vi "move2shoot Controller.vi"(8 "error in":errorcluster) -> ()   [LabVIEW 2015]
doc: "This VI executes continuously carrying out the current operation and responding to updates or new operations. It will often contain the timing or control code that is difficult to place directly in TeleOp. This VI generally opens all sensors and motors and isolates the rest of the robot code from knowing how the operations are carried out."
uses:
  move2shoot Setpoints.ctl
  move2shoot Operations.ctl
  <vilib>/Rock Robotics/WPI/SafetyOutput/WPI_SafetyOutputConfigMenu.ctl
  <vilib>/Rock Robotics/SystemInterfaces/AI/FPGA_AIChannel.ctl
  <vilib>/Rock Robotics/WPI/MotorControl/WPI_MotorControlOpenCANTalonSRX.vi
  Vision/distance.vi
  <vilib>/addons/control/pid/pid.llb/PID (DBL).vi
  <vilib>/Rock Robotics/Network Tables/NT Write Boolean.vi
  <vilib>/addons/control/pid/NI_PID_pid.lvlib
panel:
  out "Waveform Chart":dbl(graph)
  out "Encoder pos":dbl
  out "Current\nCmd":string
  # "Tip: It may be helpful to observe inputs and sensor values.\nYou may also want to display tuning or debugging controls."
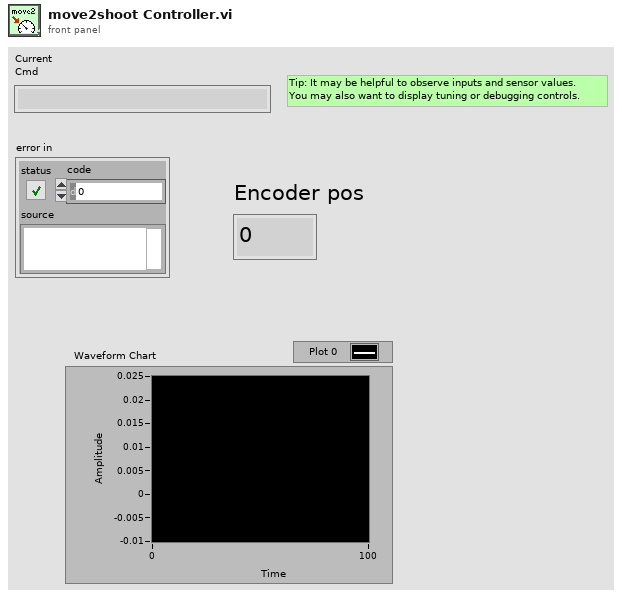
[diagram p1: front panel]
types:
  T1 = typedef "FPGA_AIChannel.ctl" = enum8{"AI 0", "AI 1", "AI 2", "AI 3", "AI MXP 0", "AI MXP 1", "AI MXP 2", "AI MXP 3", "Invalid"}
  T2 = typedef "WPI_SafetyOutputConfigMenu.ctl" = enum16{"Enable", "Disable"}
  T3 = typedef "move2shoot Setpoints.ctl" = cluster{"Operation":T4, "Setpoint":dbl, "Duration":dbl}
  T4 = typedef "move2shoot Operations.ctl" = enum16{"Reserve", "Read Current", "Immediate", "move2shoot", "go2spot"}
  T5 = typedef "WPI_MotorControlDeviceRef.ctl" = cluster{"DeviceStatus":errorcluster, "Type":T6, "PWM":cluster{"PWM Channel":T7, "DeadBand":T8}, "CAN":cluster{"Device Number":u8, "Control Mode":T9, "Semaphore":T10, "Max Vout":dbl, "TalonSRX Control Mode":T11}, "Invert":bool}
  T6 = typedef "WPI_MotorControlType.ctl" = enum16{"PWM", "CAN", "CANTalonSRX"}
  T7 = typedef "FPGA_DIOPWMChannel.ctl" = enum8{"PWM 0", "PWM 1", "PWM 2", "PWM 3", "PWM 4", "PWM 5", "PWM 6", "PWM 7", "PWM 8", "PWM 9", "PWM MXP 0", "PWM MXP 1", "PWM MXP 2", "PWM MXP 3", "PWM MXP 4", "PWM MXP 5", "PWM MXP 6", "PWM MXP 7", "PWM MXP 8", "PWM MXP 9", "Invalid"}
  T8 = typedef "WPI_PWMDeadband.ctl" = cluster{"Name":string, "maxPositivePwm":i32, "minPositivePwm":i32, "centerPwm":i32, "maxNegativePwm":i32, "minNegativePwm":i32, "angularRange":u16}
  T9 = typedef "WPI_CANJaguar_ControlMode.ctl" = enum8{"Percent VBus", "Current", "Speed", "Position", "Voltage"}
  T10 = typedef "Semaphore RefNum" = refnum<k1>
  T11 = typedef "WPI_CANTalonSRX_APIControlMode.ctl" = enum8{"Percent VBus", "Speed", "Position", "Slave", "Unchanged / Invalid", "Voltage Compensation", "Current", "Motion Profile"}
  T12 = typedef "WPI_PotentiometerDevRef.ctl" = cluster{"DevStatus":errorcluster, "Analog Channel":T1, "Invert Output":bool}
  T13 = typedef "Command Status Info.ctl" = cluster{"Name":string, "Status":T14, "notifier out":T15}
  T14 = typedef "Completion Status.ctl" = enum16{"Successful", "Aborted", "Incomplete"}
  T15 = typedef "Completion Notifier.ctl" = refnum<notifier>
  T16 = cluster{"Default Command":T3, "Command Timing":cluster{"Start Time (ms)":u32, "Iterations":i32}, "Command Arguments":cluster{"Command Info":T13, "Description":string, "Default Command":T3, "notifier out":refnum<notifier>, "Subsystem Name":string}}
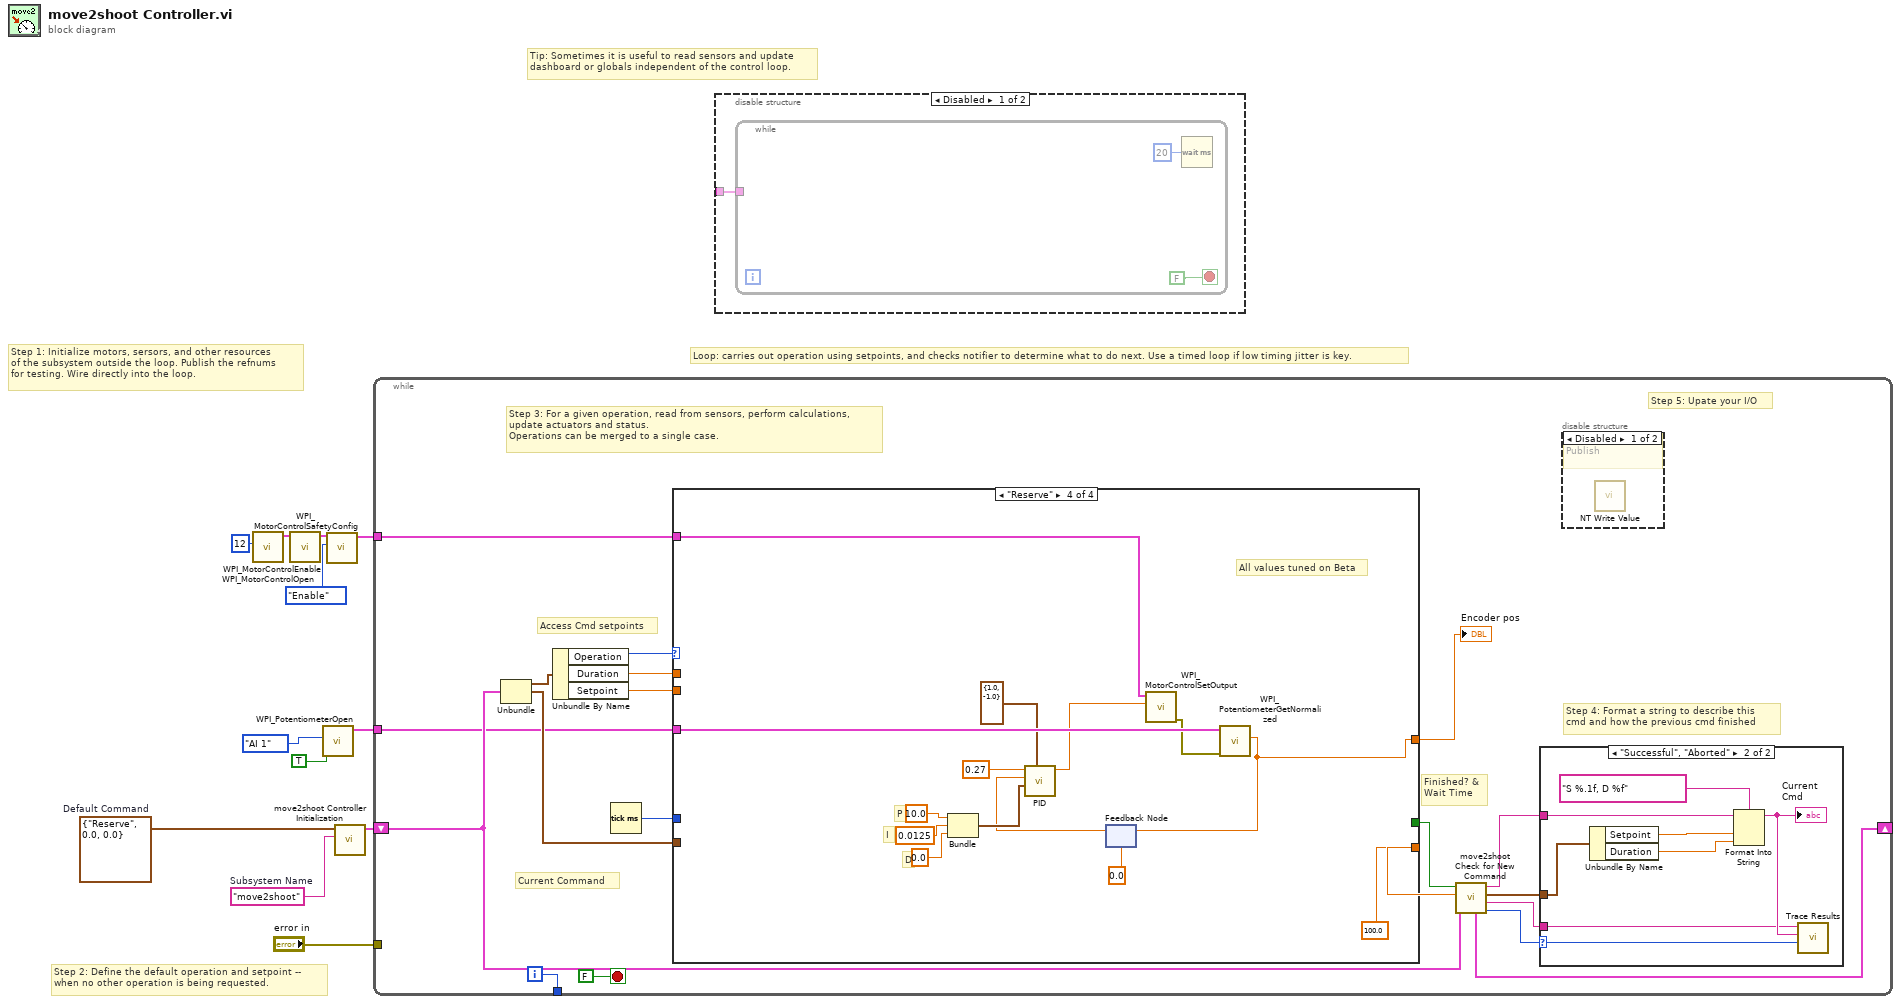
[diagram p0: block diagram]
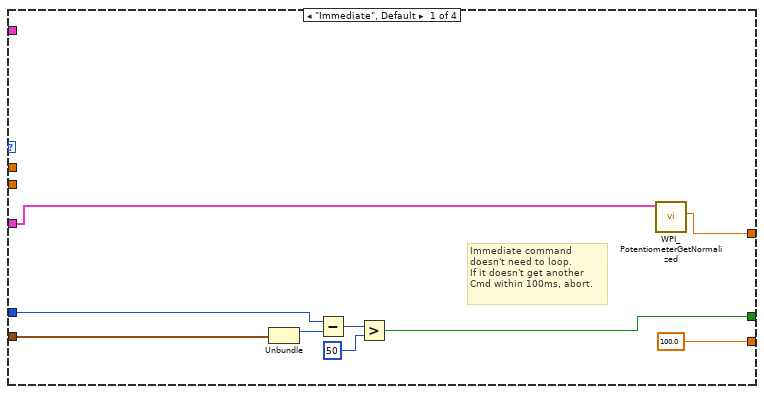
[diagram p5: hidden frame]
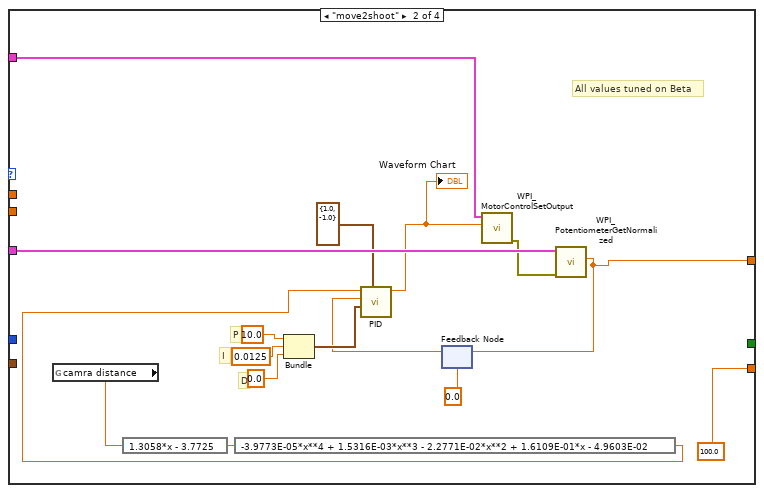
[diagram p6: hidden frame]
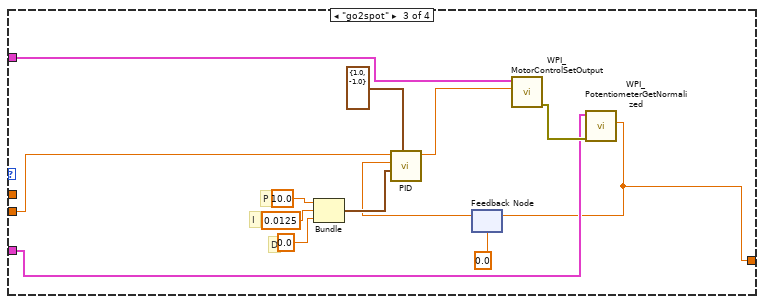
[diagram p7: hidden frame]
diagram:
  w9 = T3 {"Operation"=enum."Reserve", "Setpoint"=0.0, "Duration"=0.0}  # Default Command
  w10 = "move2shoot"  # Subsystem Name
  # "Tip: Sometimes it is useful to read sensors and update\ndashboard or globals independent of the control loop."
  # "Step 2: Define the default operation and setpoint --\nwhen no other operation is being requested."
  # "Step 1: Initialize motors, sersors, and other resources\nof the subsystem outside the loop. Publish the refnums\nfor testing. Wire directly into the loop."
  # "Loop: carries out operation using setpoints, and checks notifier to determine what to do next. Use a timed loop if low timing jitter is key."
  n1 = call-poly <vilib>:"WPI_MotorControlOpen.vi"("Device Number"=u8 12) -> ("MotorControlDeviceRef"=w6:T5)  [unwired: 9 in, 1 out]
  n2 = call <vilib>:"WPI_MotorControlEnable.vi"("CAN MotorDevRef"=w6) -> ("CAN MotorDevRef"=w7:T5)  [unwired: 9 in, 1 out]
  n3 = call <vilib>:"WPI_PotentiometerOpen.vi"("Invert Output"=TRUE, "Analog Channel"=FPGA_AIChannel."AI 1") -> ("PotDevRef"=w1:T12)  [unwired: 8 in, 1 out]
  n4 = call <vilib>:"WPI_MotorControlSafetyConfig.vi"("mode"=WPI_SafetyOutputConfigMenu."Enable", "MotorControlDevRef"=w7) -> ("MotorControlDevRef"=w4:T5)  [unwired: 8 in, 1 out]
  n5 = call "move2shoot Controller Initialization.vi"("Subsystem Name"=w10, "Default Command"=w9) -> ("Command Info"=w11:T16)  [unwired: 9 in]
  n6 = while {
    shift-right: [w22] -> _
    shift-left: w11 -> [w23]
    tunnel: [w30] -> _
    tunnel: "error in" -> [_]
    tunnel: w4 -> [w15]
    tunnel: w1 -> [w14]
    i -> [w30]
    stop <- FALSE stop-if-true
    # "Step 5: Upate your I/O"
    # "Step 4: Format a string to describe this\ncmd and how the previous cmd finished"
    # "Current Command"
    # "Access Cmd setpoints"
    # "Finished? &\nWait Time"
    # "Step 3: For a given operation, read from sensors, perform calculations,\nupdate actuators and status.\nOperations can be merged to a single case."
    n7 = Unbundle(w23) -> ("Default Command"=w29:T3, "Command Timing"=w25:cluster{"Start Time (ms)":u32, "Iterations":i32})  [unwired: 1 out]
    n8 = Unbundle By Name(w29) -> ("Operation"=w28:T4, "Duration"=w27:dbl, "Setpoint"=w24:dbl)
    n9 = Tick Count (ms)() -> (millisecond timer value=w26:u32)
    n10 = case shown="\"Reserve\"" w28 {
      tunnel: [100.0 100.0 _ 100.0] -> w20
      tunnel: [w42 _ _ _] -> w21
      tunnel: w25 -> [w44 _ _ _]
      tunnel: w27 -> [_ _ _ _]
      tunnel: w26 -> [w43 _ _ _]
      tunnel: w24 -> [_ _ w66 _]
      tunnel: w15 -> [_ w63 w68 w90]
      tunnel: w14 -> [w40 w62 w67 w89]
      tunnel: [w41 w50 w65 w78] -> w13
      frame "Immediate", Default {
        # "Immediate command\ndoesn't need to loop.\nIf it doesn't get another\nCmd within 100ms, abort."
        n11 = Unbundle(w44) -> ("Start Time (ms)"=w47:u32)  [unwired: 1 out]
        n12 = Subtract(x=w43, y=w47) -> (x-y=w46:u32)
        n13 = Greater?(x=w46, y=u8 50 ("Left Motor")) -> (0:w42:bool)
        n14 = call <vilib>:"WPI_PotentiometerGetNormalized.vi"("PotDevRef"=w40) -> ("Normalized Value"=w41:dbl)  [unwired: 8 in, 2 out]
      }
      frame "move2shoot" {
        # "All values tuned on Beta"
        # "D"
        # "I"
        # "P"
        n15 = global read "distance.vi" "camra distance"() -> (w52:dbl)
        n16 = expression code="1.3058*x - 3.7725"(w52) -> (w51:dbl)
        n17 = expression code="-3.9773E-05*x**4 + 1.5316E-03*x**3 - 2.2771E-02*x**2 + 1.6109E-01*x - 4.9603E-02"(w51) -> (w49:dbl)
        n18 = Bundle(10.0, 0.0125, 0.0) -> (w61:cluster{dbl, dbl, dbl})  [unwired: 1 in]
        n19 = feedback #1(0.0 ("Normalized Value")) -> (w57:dbl)
        n20 = call-poly <vilib>:"PID.vi"("output range"=cluster{"output high":dbl, "output low":dbl} {"output high"=1.0, "output low"=-1.0}, "PID gains"=w61, "process variable"=w57, "setpoint"=w49) -> ("output"=w58:dbl)  [unwired: 6 in, 1 out]
        "Waveform Chart" <- w58
        n21 = call <vilib>:"WPI_MotorControlSetOutput.vi"("Output"=w58, "MotorControlDevRef"=w63) -> ("error out"=w60:errorcluster)  [unwired: 7 in, 2 out]
        n22 = call <vilib>:"WPI_PotentiometerGetNormalized.vi"("error in"=w60, "PotDevRef"=w62) -> ("Normalized Value"=w50:dbl)  [unwired: 7 in, 2 out]
        n23 = feedback-in #1(w50) -> ()
      }
      frame "go2spot" {
        # "D"
        # "I"
        # "P"
        n24 = Bundle(10.0, 0.0125, 0.0) -> (w77:cluster{dbl, dbl, dbl})  [unwired: 1 in]
        n25 = feedback #2(0.0 ("Normalized Value")) -> (w73:dbl)
        n26 = call-poly <vilib>:"PID.vi"("output range"=cluster{"output high":dbl, "output low":dbl} {"output high"=1.0, "output low"=-1.0}, "PID gains"=w77, "process variable"=w73, "setpoint"=w66) -> ("output"=w74:dbl)  [unwired: 6 in, 1 out]
        n27 = call <vilib>:"WPI_MotorControlSetOutput.vi"("Output"=w74, "MotorControlDevRef"=w68) -> ("error out"=w76:errorcluster)  [unwired: 7 in, 2 out]
        n28 = call <vilib>:"WPI_PotentiometerGetNormalized.vi"("error in"=w76, "PotDevRef"=w67) -> ("Normalized Value"=w65:dbl)  [unwired: 7 in, 2 out]
        n29 = feedback-in #2(w65) -> ()
      }
      frame "Reserve" {
        # "All values tuned on Beta"
        # "D"
        # "I"
        # "P"
        n30 = Bundle(10.0, 0.0125, 0.0) -> (w88:cluster{dbl, dbl, dbl})  [unwired: 1 in]
        n31 = feedback #3(0.0 ("Normalized Value")) -> (w84:dbl)
        n32 = call-poly <vilib>:"PID.vi"("output range"=cluster{"output high":dbl, "output low":dbl} {"output high"=1.0, "output low"=-1.0}, "PID gains"=w88, "process variable"=w84, "setpoint"=0.27) -> ("output"=w85:dbl)  [unwired: 6 in, 1 out]
        n33 = call <vilib>:"WPI_MotorControlSetOutput.vi"("Output"=w85, "MotorControlDevRef"=w90) -> ("error out"=w87:errorcluster)  [unwired: 7 in, 2 out]
        n34 = call <vilib>:"WPI_PotentiometerGetNormalized.vi"("error in"=w87, "PotDevRef"=w89) -> ("Normalized Value"=w78:dbl)  [unwired: 7 in, 2 out]
        n35 = feedback-in #3(w78) -> ()
      }
    }
    "Encoder pos" <- w13
    n36 = call "move2shoot Check for New Command.vi"("Current Command"=w23, "Wait time (ms)"=w20, "Finished?"=w21) -> ("Completion"=w16:T14, "Subsystem Name"=w17:string, "Current Command"=w18:T3, "Initial Trace String"=w19:string, "NextCommand"=w22:T16)  [unwired: 4 in]
    n37 = case shown="\"Successful\", \"Aborted\"" w16 {
      selector: w16 -> [_ w39]
      tunnel: w19 -> [_ w35]
      tunnel: w18 -> [_ w36]
      tunnel: w17 -> [_ w32]
      frame "Incomplete", Default {
        # "Continuing current command"
      }
      frame "Successful", "Aborted" {
        # "Report and setup for next command"
        n38 = Unbundle By Name(w36) -> ("Setpoint"=w38:dbl, "Duration"=w33:dbl)
        n39 = Format Into String(format string="S %.1f, D %f", initial string=w35, w38, w33) -> (resulting string=w34:string)  [unwired: 1 in, 1 out]
        "Current\nCmd" <- w34
        n40 = call <vilib>:"Trace Results.vi"("Status of previous command"=w39, "Description"=w34, "Subsystem"=w32) -> ()  [unwired: 9 in]
      }
    }
    n41 = disable-structure shown="Disabled" {
      frame Disabled {
        # "Publish"
        n42 = call-poly <vilib>:"NT Write Value.vi"() -> ()  [unwired: 11 in, 1 out]
      }
      frame Enabled {
      }
    }
  }
  n43 = disable-structure shown="Disabled" {
    disable-tunnel: _ -> [w92 _]
    frame Disabled {
      n44 = while {
        tunnel: w92 -> [_]
        stop <- FALSE stop-if-true
        n45 = Wait (ms)(milliseconds to wait=u32 20) -> ()  [unwired: 1 out]
      }
    }
    frame Enabled {
    }
  }
